vi "CloseStreams.vi"(7 "Qbus in":refnum<class "Qbus.lvclass">, 8 "error in (no error)":errorcluster, 11 "config in":T1) -> (0 "error out":errorcluster, 3 "config out":T1)   [LabVIEW 2017, in "CmsDataEventCreator.lvlib"]
uses:
  <vilib>/addons/InsightCM/Devices/Shared/Cms/CmsDataEventCreator/CmsDataEventCreator.lvlib
  <vilib>/addons/InsightCM/Devices/Shared/Cms/CmsDataEventCreator/controls/config.ctl
  <vilib>/addons/Qbus/Qbus.lvclass
  <vilib>/addons/InsightCM/MessageBus/MessageLibrary/DataStorage/controls/DataStorageCloseStreamRoutedMessageBody.ctl
  <vilib>/addons/InsightCM/Devices/Shared/Common/ServerComm/ServerComm.lvlib
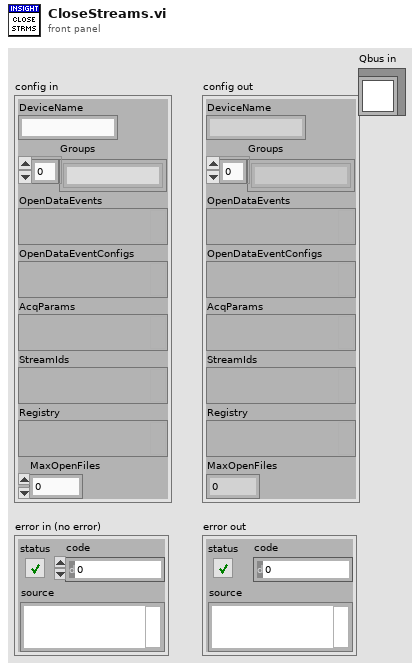
[diagram p1: front panel]
types:
  T1 = typedef "CmsDataEventCreator.lvlib/config.ctl" = cluster{"DeviceName":string, "Groups":string[], "OpenDataEvents":variant, "OpenDataEventConfigs":variant, "AcqParams":variant, "StreamIds":variant, "Registry":variant, "MaxOpenFiles":i32}
  T2 = typedef "DataStorageCloseStreamRoutedMessageBody.ctl" = cluster{"StreamId":string}
  T3 = typedef "Message.ctl" = cluster{"Header":T4, "Body":u8[]}
  T4 = typedef "MessageHeader.ctl" = cluster{"MessageName":string, "Timestamp":i64, "CorrelationId":string, "ContentType":string, "RoutingKey":string, "Properties":T5[]}
  T5 = typedef "KeyValuePair.ctl" = cluster{"Key":string, "Value":string}
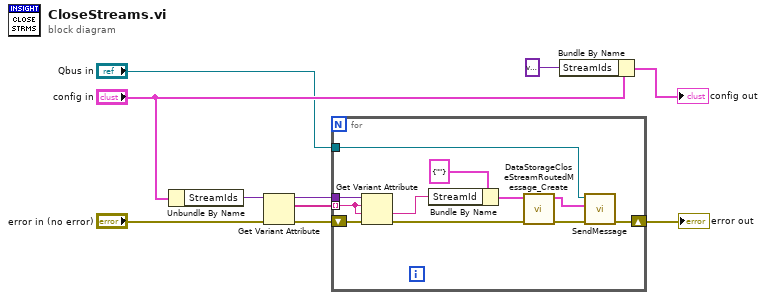
[diagram p0: block diagram]
diagram:
  n1 = Unbundle By Name("config in") -> ("StreamIds"=w10:variant)
  n2 = Get Variant Attribute(Variant=w10, error in="error in (no error)") -> (duplicate Variant=w1:variant, names=w2:string[], error out=w8:errorcluster)  [unwired: 2 in, 1 out]
  n3 = for {
    shift-right: [w19] -> w7
    shift-left: w8 -> [w15]
    tunnel: "Qbus in" -> [w21]
    tunnel: w2 -> [w12] mode=indexing
    tunnel: w1 -> [w13]
    n4 = Get Variant Attribute(Variant=w13, name=w12, default value (empty Variant)=w12, error in=w15) -> (value=w11:string, error out=w14:errorcluster)  [unwired: 2 out]
    n5 = Bundle By Name(cluster=T2 {"StreamId"=""} ("DataStorageCloseStreamRoutedMessage"), "StreamId"=w11) -> (w16:T2)
    n6 = call <vilib>:"DataStorageCloseStreamRoutedMessage_Create.vi"("error in (no error)"=w14, "DataStorageCloseStreamRoutedMessage"=w16) -> ("error out"=w18:errorcluster, "Message"=w20:T3)  [unwired: 8 in]
    n7 = call <vilib>:"SendMessage.vi"("error in (no error)"=w18, "message"=w20, "Qbus in"=w21) -> ("error out"=w19:errorcluster)  [unwired: 7 in, 1 out]
  }
  "error out" <- w7
  n8 = Bundle By Name(cluster="config in", "StreamIds"=variant) -> (→"config out":T1)
